vi "Register gRPC Methods.vi"(8 "error in (no error)":errorcluster, 11 "Template Server in":refnum<class "Manager.lvclass">) -> (0 "error out":errorcluster, 3 "Template Server out":refnum<class "Manager.lvclass">)   [LabVIEW 2021, in "CIF_Manager_server.lvlib" / "Manager.lvclass"]
uses:
  Manager.lvclass
  typeDefs/Server Internal UEs.ctl
  typeDefs/Server Internal Message.ctl
  typeDefs/Server gRPC UEs.ctl
  <vilib>/gRPC/LabVIEW gRPC Library/Server API/typeDefs/gRPCId Cluster.ctl
  <vilib>/gRPC/LabVIEW gRPC Library/Shared/grpcId.ctl
  Manager.lvclass/Manager.ctl
  <vilib>/gRPC/LabVIEW gRPC Library/grpc-lvsupport-release.lvlib
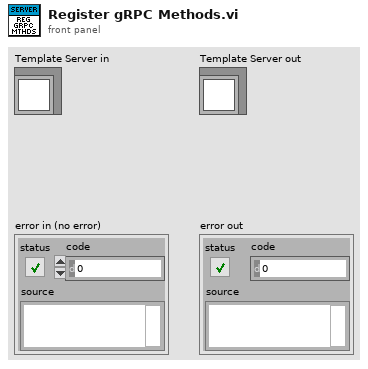
[diagram p1: front panel]
types:
  T1 = typedef "CIF_Manager_server.lvlib/Manager.lvclass/Server gRPC UEs.ctl" = cluster{"Manager LoadPlugin gRPC UE":refnum<user-event>, "Manager RegisterPlugin gRPC UE":refnum<user-event>, "Manager UnregisterPlugin gRPC UE":refnum<user-event>, "Manager QueryPluginTypes gRPC UE":refnum<user-event>, "Manager AbortPlugin gRPC UE":refnum<user-event>, "Manager UnloadAllPlugins gRPC UE":refnum<user-event>, "Manager Destroy gRPC UE":refnum<user-event>, "Manager Ping gRPC UE":refnum<user-event>, "Manager QueryErrors gRPC UE":refnum<user-event>, "Manager QueryConfig gRPC UE":refnum<user-event>, "Manager QueryInfo gRPC UE":refnum<user-event>, "Manager ResetErrorIndex gRPC UE":refnum<user-event>, "Manager ResetConfigIndex gRPC UE":refnum<user-event>, "Manager ResetInfoIndex gRPC UE":refnum<user-event>, "Manager QueryPluginInfo gRPC UE":refnum<user-event>, "Manager QueryPlugin gRPC UE":refnum<user-event>}
  T2 = typedef "CIF_Manager_server.lvlib/Manager.lvclass/Server Internal UEs.ctl" = cluster{"Manager LoadPlugin Internal UE":refnum<user-event>, "Manager RegisterPlugin Internal UE":refnum<user-event>, "Manager UnregisterPlugin Internal UE":refnum<user-event>, "Manager QueryPluginTypes Internal UE":refnum<user-event>, "Manager AbortPlugin Internal UE":refnum<user-event>, "Manager UnloadAllPlugins Internal UE":refnum<user-event>, "Manager Destroy Internal UE":refnum<user-event>, "Manager Ping Internal UE":refnum<user-event>, "Manager QueryErrors Internal UE":refnum<user-event>, "Manager QueryConfig Internal UE":refnum<user-event>, "Manager QueryInfo Internal UE":refnum<user-event>, "Manager ResetErrorIndex Internal UE":refnum<user-event>, "Manager ResetConfigIndex Internal UE":refnum<user-event>, "Manager ResetInfoIndex Internal UE":refnum<user-event>, "Manager QueryPluginInfo Internal UE":refnum<user-event>, "Manager QueryPlugin Internal UE":refnum<user-event>}
  T3 = typedef "grpc-lvsupport-release.lvlib/grpcId.ctl" = u64
  T4 = typedef "CIF_Manager_server.lvlib/Manager.lvclass/Server Internal Message UE.ctl" = refnum<user-event>
  T5 = typedef "grpc-lvsupport-release.lvlib/gRPCId Cluster UE.ctl" = refnum<user-event>
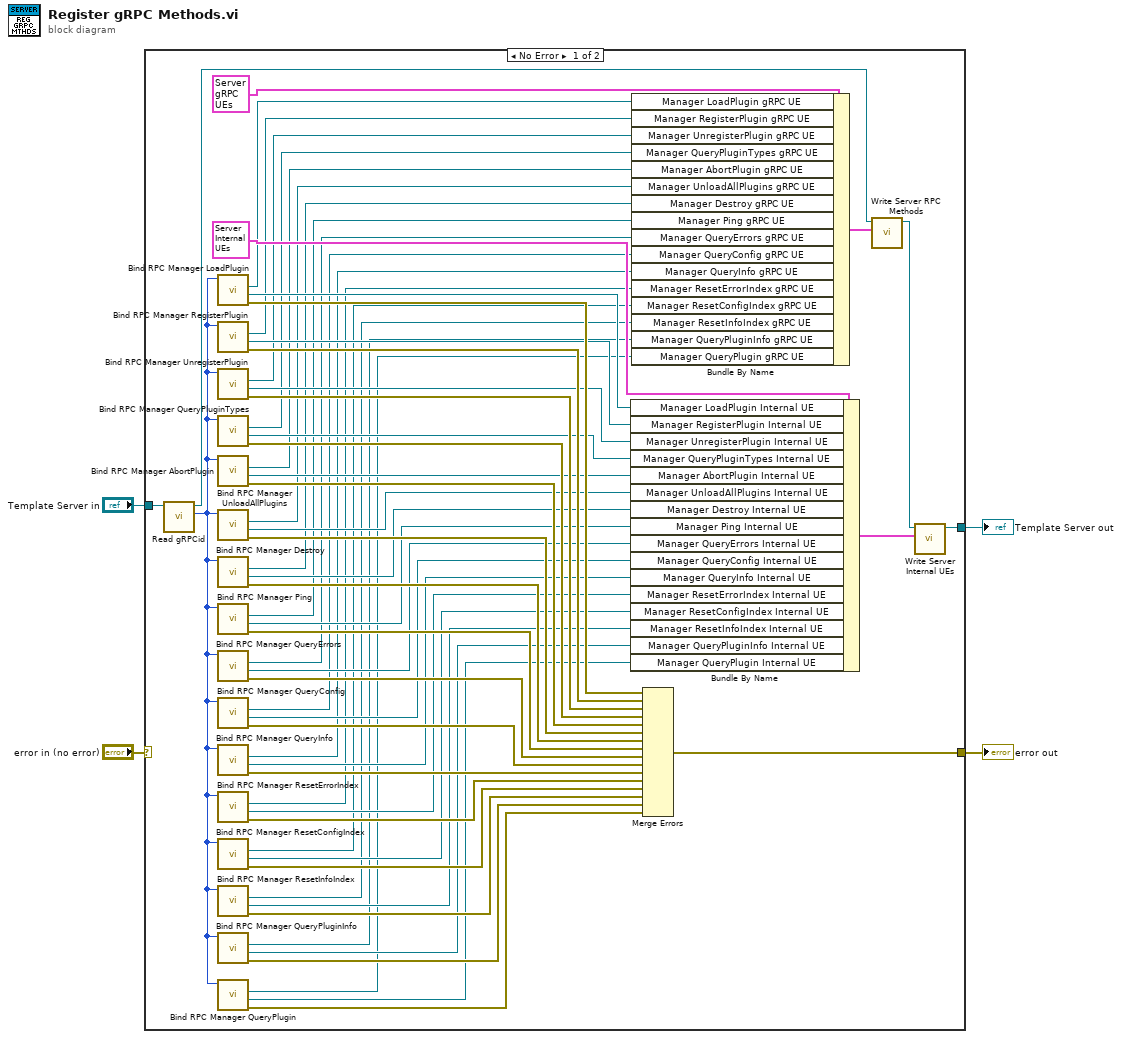
[diagram p0: block diagram]
diagram:
  n1 = case shown="No Error" "error in (no error)" {
    selector: "error in (no error)" -> [_ w63]
    tunnel: "Template Server in" -> [w54 w64]
    tunnel: [w62 w63] -> w3
    tunnel: [w61 w64] -> w2
    frame No Error {
      n2 = call-dynamic "Read gRPCid.vi"("iService in"=w54) -> ("gRPCid"=w53:T3, "iService out"=w55:refnum<class "Manager.lvclass">)  [unwired: 8 in, 1 out]
      n3 = call "Bind RPC Manager LoadPlugin.vi"("gRPCid server in"=w53) -> ("error out"=w52:errorcluster, "Manager LoadPlugin Internal UE"=w50:T4, "Manager LoadPlugin gRPC UE"=w51:T5)  [unwired: 7 in, 1 out]
      n4 = call "Bind RPC Manager RegisterPlugin.vi"("gRPCid server in"=w53) -> ("error out"=w49:errorcluster, "Manager RegisterPlugin Internal UE"=w47:T4, "Manager RegisterPlugin gRPC UE"=w48:T5)  [unwired: 7 in, 1 out]
      n5 = call "Bind RPC Manager UnregisterPlugin.vi"("gRPCid server in"=w53) -> ("error out"=w46:errorcluster, "Manager UnregisterPlugin Internal UE"=w44:T4, "Manager UnregisterPlugin gRPC UE"=w45:T5)  [unwired: 7 in, 1 out]
      n6 = call "Bind RPC Manager QueryPluginTypes.vi"("gRPCid server in"=w53) -> ("error out"=w43:errorcluster, "Manager QueryPluginTypes Internal UE"=w41:T4, "Manager QueryPluginTypes gRPC UE"=w42:T5)  [unwired: 7 in, 1 out]
      n7 = call "Bind RPC Manager AbortPlugin.vi"("gRPCid server in"=w53) -> ("error out"=w40:errorcluster, "Manager AbortPlugin Internal UE"=w38:T4, "Manager AbortPlugin gRPC UE"=w39:T5)  [unwired: 7 in, 1 out]
      n8 = call "Bind RPC Manager UnloadAllPlugins.vi"("gRPCid server in"=w53) -> ("error out"=w37:errorcluster, "Manager UnloadAllPlugins Internal UE"=w35:T4, "Manager UnloadAllPlugins gRPC UE"=w36:T5)  [unwired: 7 in, 1 out]
      n9 = call "Bind RPC Manager Destroy.vi"("gRPCid server in"=w53) -> ("error out"=w34:errorcluster, "Manager Destroy Internal UE"=w32:T4, "Manager Destroy gRPC UE"=w33:T5)  [unwired: 7 in, 1 out]
      n10 = call "Bind RPC Manager Ping.vi"("gRPCid server in"=w53) -> ("error out"=w31:errorcluster, "Manager Ping Internal UE"=w29:T4, "Manager Ping gRPC UE"=w30:T5)  [unwired: 7 in, 1 out]
      n11 = call "Bind RPC Manager QueryErrors.vi"("gRPCid server in"=w53) -> ("error out"=w28:errorcluster, "Manager QueryErrors Internal UE"=w26:T4, "Manager QueryErrors gRPC UE"=w27:T5)  [unwired: 7 in, 1 out]
      n12 = call "Bind RPC Manager QueryConfig.vi"("gRPCid server in"=w53) -> ("error out"=w25:errorcluster, "Manager QueryConfig Internal UE"=w23:T4, "Manager QueryConfig gRPC UE"=w24:T5)  [unwired: 7 in, 1 out]
      n13 = call "Bind RPC Manager QueryInfo.vi"("gRPCid server in"=w53) -> ("error out"=w22:errorcluster, "Manager QueryInfo Internal UE"=w20:T4, "Manager QueryInfo gRPC UE"=w21:T5)  [unwired: 7 in, 1 out]
      n14 = call "Bind RPC Manager ResetErrorIndex.vi"("gRPCid server in"=w53) -> ("error out"=w19:errorcluster, "Manager ResetErrorIndex Internal UE"=w17:T4, "Manager ResetErrorIndex gRPC UE"=w18:T5)  [unwired: 7 in, 1 out]
      n15 = call "Bind RPC Manager ResetConfigIndex.vi"("gRPCid server in"=w53) -> ("error out"=w16:errorcluster, "Manager ResetConfigIndex Internal UE"=w14:T4, "Manager ResetConfigIndex gRPC UE"=w15:T5)  [unwired: 7 in, 1 out]
      n16 = call "Bind RPC Manager ResetInfoIndex.vi"("gRPCid server in"=w53) -> ("error out"=w13:errorcluster, "Manager ResetInfoIndex Internal UE"=w11:T4, "Manager ResetInfoIndex gRPC UE"=w12:T5)  [unwired: 7 in, 1 out]
      n17 = call "Bind RPC Manager QueryPluginInfo.vi"("gRPCid server in"=w53) -> ("error out"=w10:errorcluster, "Manager QueryPluginInfo Internal UE"=w8:T4, "Manager QueryPluginInfo gRPC UE"=w9:T5)  [unwired: 7 in, 1 out]
      n18 = call "Bind RPC Manager QueryPlugin.vi"("gRPCid server in"=w53) -> ("error out"=w7:errorcluster, "Manager QueryPlugin Internal UE"=w5:T4, "Manager QueryPlugin gRPC UE"=w6:T5)  [unwired: 7 in, 1 out]
      n19 = Bundle By Name ("Bundle Internal UEs")(cluster=T2 {"Manager LoadPlugin Internal UE"=refnum, "Manager RegisterPlugin Internal UE"=refnum, "Manager UnregisterPlugin Internal UE"=refnum, "Manager QueryPluginTypes Internal UE"=refnum, "Manager AbortPlugin Internal UE"=refnum, "Manager UnloadAllPlugins Internal UE"=refnum, "Manager Destroy Internal UE"=refnum, "Manager Ping Internal UE"=refnum, "Manager QueryErrors Internal UE"=refnum, "Manager QueryConfig Internal UE"=refnum, "Manager QueryInfo Internal UE"=refnum, "Manager ResetErrorIndex Internal UE"=refnum, "Manager ResetConfigIndex Internal UE"=refnum, "Manager ResetInfoIndex Internal UE"=refnum, "Manager QueryPluginInfo Internal UE"=refnum, "Manager QueryPlugin Internal UE"=refnum} ("Server Internal UEs"), "Manager LoadPlugin Internal UE"=w50, "Manager RegisterPlugin Internal UE"=w47, "Manager UnregisterPlugin Internal UE"=w44, "Manager QueryPluginTypes Internal UE"=w41, "Manager AbortPlugin Internal UE"=w38, "Manager UnloadAllPlugins Internal UE"=w35, "Manager Destroy Internal UE"=w32, "Manager Ping Internal UE"=w29, "Manager QueryErrors Internal UE"=w26, "Manager QueryConfig Internal UE"=w23, "Manager QueryInfo Internal UE"=w20, "Manager ResetErrorIndex Internal UE"=w17, "Manager ResetConfigIndex Internal UE"=w14, "Manager ResetInfoIndex Internal UE"=w11, "Manager QueryPluginInfo Internal UE"=w8, "Manager QueryPlugin Internal UE"=w5) -> (w60:T2)
      n20 = Bundle By Name ("Bundle gRPC UEs")(cluster=T1 {"Manager LoadPlugin gRPC UE"=refnum, "Manager RegisterPlugin gRPC UE"=refnum, "Manager UnregisterPlugin gRPC UE"=refnum, "Manager QueryPluginTypes gRPC UE"=refnum, "Manager AbortPlugin gRPC UE"=refnum, "Manager UnloadAllPlugins gRPC UE"=refnum, "Manager Destroy gRPC UE"=refnum, "Manager Ping gRPC UE"=refnum, "Manager QueryErrors gRPC UE"=refnum, "Manager QueryConfig gRPC UE"=refnum, "Manager QueryInfo gRPC UE"=refnum, "Manager ResetErrorIndex gRPC UE"=refnum, "Manager ResetConfigIndex gRPC UE"=refnum, "Manager ResetInfoIndex gRPC UE"=refnum, "Manager QueryPluginInfo gRPC UE"=refnum, "Manager QueryPlugin gRPC UE"=refnum} ("gRPC Server Method Events"), "Manager LoadPlugin gRPC UE"=w51, "Manager RegisterPlugin gRPC UE"=w48, "Manager UnregisterPlugin gRPC UE"=w45, "Manager QueryPluginTypes gRPC UE"=w42, "Manager AbortPlugin gRPC UE"=w39, "Manager UnloadAllPlugins gRPC UE"=w36, "Manager Destroy gRPC UE"=w33, "Manager Ping gRPC UE"=w30, "Manager QueryErrors gRPC UE"=w27, "Manager QueryConfig gRPC UE"=w24, "Manager QueryInfo gRPC UE"=w21, "Manager ResetErrorIndex gRPC UE"=w18, "Manager ResetConfigIndex gRPC UE"=w15, "Manager ResetInfoIndex gRPC UE"=w12, "Manager QueryPluginInfo gRPC UE"=w9, "Manager QueryPlugin gRPC UE"=w6) -> (w57:T1)
      n21 = Merge Errors(w52, w49, w46, w43, w40, w37, w34, w31, w28, w25, w22, w19, w16, w13, w10, w7) -> (w62:errorcluster)
      n22 = call "Write Server RPC Methods.vi"("Server RPC Methods"=w57, "SignalGeneratorService in"=w55) -> ("SignalGeneratorService out"=w58:refnum<class "Manager.lvclass">)  [unwired: 8 in, 1 out]
      n23 = call "Write Server Internal UEs.vi"("Server Internal UEs"=w60, "SignalGeneratorService in"=w58) -> ("SignalGeneratorService out"=w61:refnum<class "Manager.lvclass">)  [unwired: 8 in, 1 out]
    }
    frame Error {
    }
  }
  "error out" <- w3
  "Template Server out" <- w2
